vi "Initialize EtherCAT youBot Platform.vi"(8 "error in (no error)":errorcluster, 11 "arm slave infos":T1[](array[typedef]) {"nodeAddr" format="%.0x"}) -> (0 "error out":errorcluster, 3 "KUKA youBot platform_EtherCAT out":refnum<class "NI_Robotics_KUKA youBot Platform_EtherCAT.lvclass">)   [LabVIEW 2017, in "NI_Robotics_KUKA youBot Host.lvlib" / "NI_Robotics_KUKA youBot Platform_EtherCAT.lvclass"]
uses:
  <vilib>/robotics/KUKA youBot/Basic Device/Mobile Platform EtherCAT/NI_Robotics_KUKA youBot Platform_EtherCAT.lvclass
  c:/Program Files (x86)/National Instruments/LabVIEW 2017/vi.lib/robotics/KUKA youBot/Basic Device/Mobile Platform/NI_Robotics_KUKA youBot Platform.lvclass
  <vilib>/robotics/KUKA youBot/EtherCAT/Motor Slave Info.ctl
  <vilib>/robotics/KUKA youBot/EtherCAT/LowLevel/Mater Handler.ctl
  <vilib>/robotics/KUKA youBot/Motor/Wheel Motor EtherCAT/NI_Robotics_KUKA youBot Wheel Motor_EtherCAT.lvclass
  c:/Program Files (x86)/National Instruments/LabVIEW 2017/vi.lib/robotics/KUKA youBot/Motor/Wheel Motor/NI_Robotics_KUKA youBot Wheel Motor.lvclass
  <vilib>/robotics/KUKA youBot/Basic Device/Mobile Platform/NI_Robotics_KUKA youBot Platform.lvclass
  <vilib>/robotics/KUKA youBot/NI_Robotics_KUKA youBot Host.lvlib
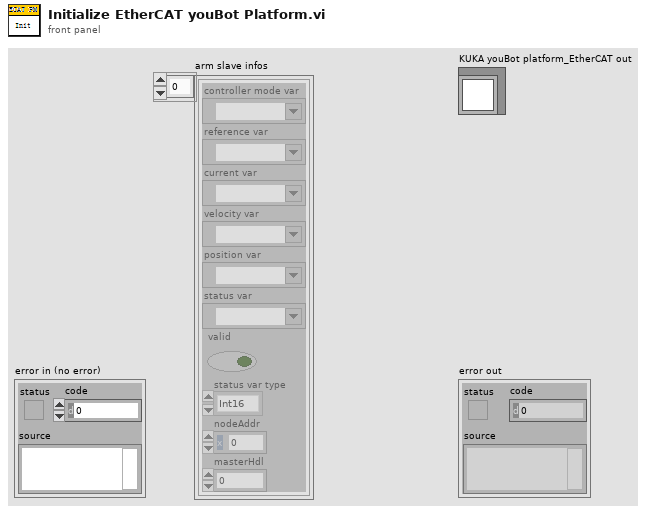
[diagram p1: front panel]
types:
  T1 = typedef "NI_Robotics_KUKA youBot Host.lvlib/Motor Slave Info.ctl" = cluster{"controller mode var":refnum<k21>, "reference var":refnum<k21>, "current var":refnum<k21>, "velocity var":refnum<k21>, "position var":refnum<k21>, "status var":refnum<k21>, "valid":bool, "status var type":enum16{"Int16", "Int32"}, "nodeAddr":u16, "masterHdl":T2}
  T2 = typedef "NI_Robotics_KUKA youBot Host.lvlib/Mater Handler.ctl" = i32
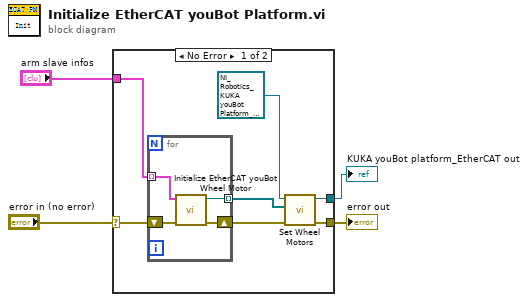
[diagram p0: block diagram]
diagram:
  n1 = case shown="No Error" "error in (no error)" {
    selector: "error in (no error)" -> [w10 w16]
    tunnel: [w7 w16] -> w3
    tunnel: "arm slave infos" -> [w11 _]
    tunnel: [w5 _] -> w1
    frame No Error {
      n2 = for {
        tunnel: w11 -> [w12] mode=indexing
        shift-right: [w14] -> w8
        shift-left: w10 -> [w15]
        tunnel: [w13] -> w6 mode=indexing
        n3 = call <vilib>:"Initialize EtherCAT youBot Wheel Motor.vi"("error in (no error)"=w15, "motor slave info in"=w12) -> ("error out"=w14:errorcluster, "KUKA youBot wheel motor_EtherCAT out"=w13:refnum<class "NI_Robotics_KUKA youBot Wheel Motor_EtherCAT.lvclass">)  [unwired: 8 in]
      }
      n4 = call <vilib>:"Set Wheel Motors.vi"("error in (no error)"=w8, "wheel motors"=w6, "KUKA youBot platform in"=refnum<class "NI_Robotics_KUKA youBot Platform_EtherCAT.lvclass"> refnum ("NI_Robotics_KUKA youBot Host.lvlib:NI_Robotics_KUKA youBot Platform_EtherCAT.lvclass")) -> ("error out"=w7:errorcluster, "KUKA youBot platform out"=w5:refnum<class "NI_Robotics_KUKA youBot Platform_EtherCAT.lvclass">)  [unwired: 7 in]
    }
    frame Error {
    }
  }
  "error out" <- w3
  "KUKA youBot platform_EtherCAT out" <- w1
